vi "SUB_SND_OUT_RCV.vi"(6 "frequency":dbl=2000.0, 7 "R Channel On OFF":dbl=1.0 format="%0.2p", 8 "L Chanel On Off":dbl=1.0 format="%0.2p", 10 "ID_用那一張音效卡做輸出":u32) -> ()   [LabVIEW 2011]
uses:
  Instance           1 23Saved   SUB_SND_OUT_RCV .vi
  <vilib>/measure/NI_MABase.lvlib
  <vilib>/Analysis/NI_AALPro.lvlib
panel:
  out "Input Frequence HZ":i32
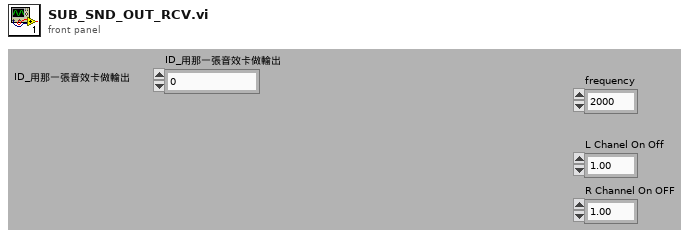
[diagram p1: front panel]
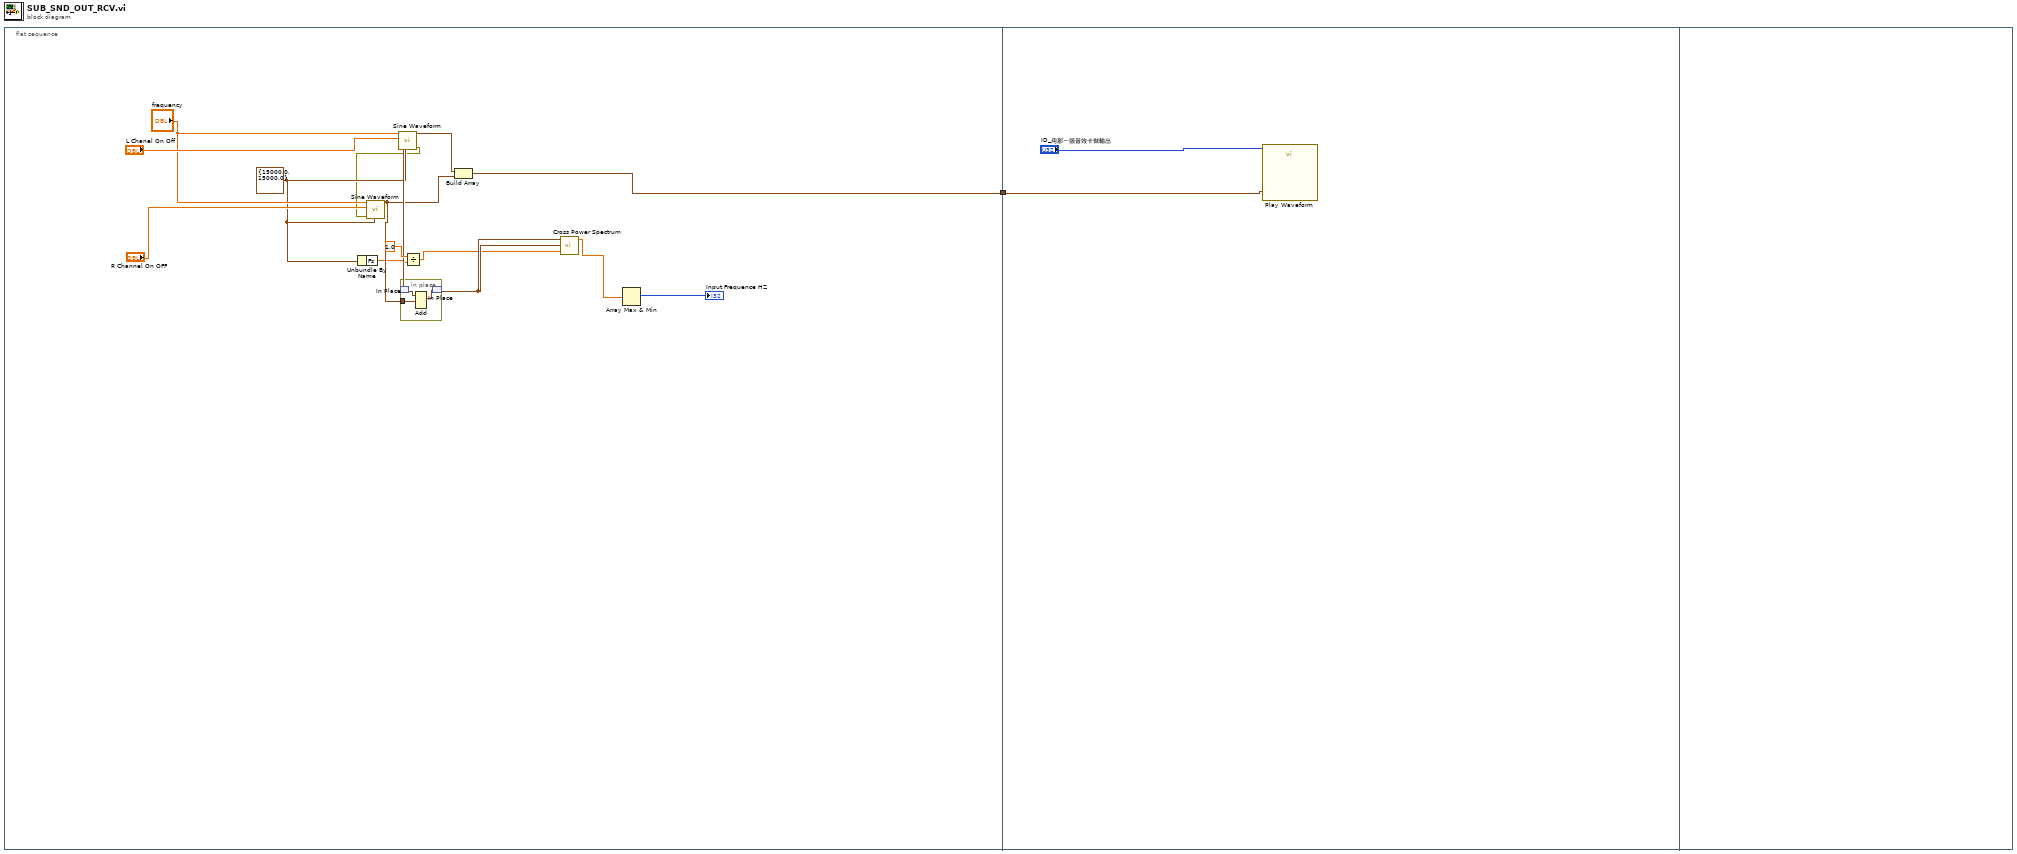
[diagram p0: block diagram]
diagram:
  n1 = flat-sequence {
    tunnel: [w3] -> w1
    tunnel: w1 -> [w20]
    frame #0 {
      w5 = cluster{"Fs":dbl, "#s":dbl} {"Fs"=15000.0, "#s"=15000.0} ("sampling info")
      n2 = Unbundle By Name(w5) -> ("Fs"=w9:dbl)
      n3 = call <vilib>:"Sine Waveform.vi"("sampling info"=w5, "amplitude"="L Chanel On Off", "frequency"="frequency") -> ("error out"=w4:errorcluster, "signal out"=w12:waveform(dbl))  [unwired: 7 in]
      n4 = call <vilib>:"Sine Waveform.vi"("sampling info"=w5, "error in (no error)"=w4, "amplitude"="R Channel On OFF", "frequency"="frequency") -> ("signal out"=w11:waveform(dbl))  [unwired: 6 in, 1 out]
      n5 = in-place {
        in-place-border: w11 -> [w17]
        n6 = in-place-match #1(w12) -> (w18:waveform(dbl))
        n7 = Add(1:w17, 2:w18) -> (0:w16:waveform(dbl))  [unwired: 1 in, 1 out]
        n8 = in-place-match #1(w16) -> (w10:waveform(dbl))
      }
      n9 = Divide(x=1.0, y=w9) -> (x/y=w2:dbl)
      n10 = Build Array(w12, w11) -> (w3:waveform(dbl)[])
      n11 = call <vilib>:"Cross Power Spectrum.vi"("dt"=w2, "Signal Y (V)"=w10, "Signal X (V)"=w10) -> ("Cross Power XY Spectrum Mag (V^2rms)"=w14:dbl[])  [unwired: 2 out]
      n12 = Array Max & Min(array=w14) -> (max index (indices)=→"Input Frequence HZ":i32)  [unwired: 3 out]
    }
    frame #1 {
      n13 = call "Play Waveform"("Device"="ID_用那一張音效卡做輸出", "Data"=w20) -> ()  [unwired: 17 in, 1 out]
    }
    frame #2 {
    }
  }
